vi "get Header Msg.vi"(9 "pseudoPdcId":i32, 10 "maxMsgLength":i32, 11 "msg":string) -> (2 "function return":i32, 3 "msg out":string)   [LabVIEW 2013, in "C37118-DLL.lvlib" / "StrongridDLL.lvlib"]
doc: "STRONGRIDIEEEC37118DLL_API int __cdecl getHeaderMsg( char* msg, int maxMsgLength, int32_t pseudoPdcId);"
uses:
  StrongridDLL.lvlib
  StrongridDLL/StrongridDLL.dll
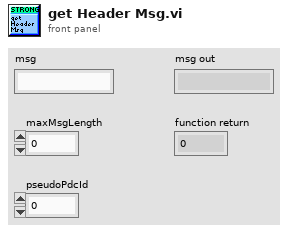
[diagram p1: front panel]
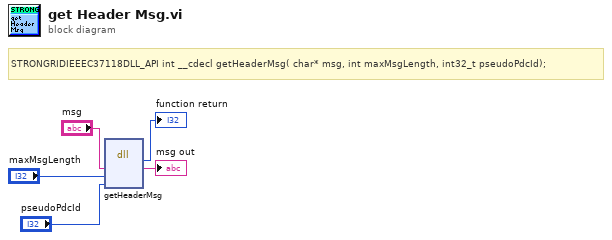
[diagram p0: block diagram]
diagram:
  # "STRONGRIDIEEEC37118DLL_API int __cdecl getHeaderMsg( char* msg, int maxMsgLength, int32_t pseudoPdcId);"
  n1 = dll-call lib="C:/dev/OSS/S3DK/builds/StrongridDLL/StrongridDLL.*" fn="getHeaderMsg"("msg"="msg", "maxMsgLength"="maxMsgLength", "pseudoPdcId"="pseudoPdcId") -> (→"function return":i32, "msg"=→"msg out":string)  [unwired: 5 in, 2 out]
